vi "Remove illegal characters fr filename.vi"(3 "Filename In":string) -> (1 "Cleaned Filename":string)   [LabVIEW 2022 SP3]
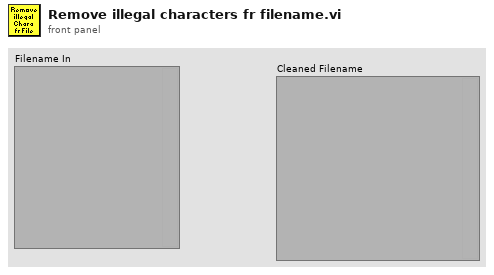
[diagram p1: front panel]
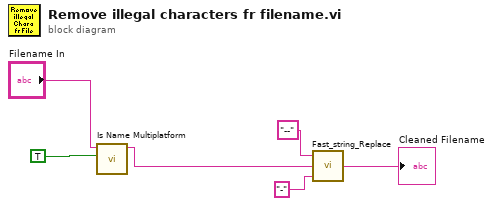
[diagram p0: block diagram]
diagram:
  n1 = call <vilib>:"Is Name Multiplatform.vi"("filename must be valid on all platforms (F)"=TRUE, "filename"="Filename In") -> ("suggested filename"=w1:string)  [unwired: 5 in, 4 out]
  n2 = call "Fast_string_Replace.vi"("Replace match with:"="-", "Input String"=w1, "matchThis"="--" ("regular expression")) -> ("Output String"=→"Cleaned Filename":string)  [unwired: 1 in, 1 out]
